vi "SQL_EDITOR_prepare_SELECT_statement.vi"(7 "nmb_of_top_rows (all)":i32, 8 "error_in":errorcluster) -> (0 "error_out":errorcluster, 3 "SELECT_statement":string)   [LabVIEW 2019]
uses:
  FGV/SQL_EDITOR_records_display/FGV_SQL_EDITOR_records_display.ctl
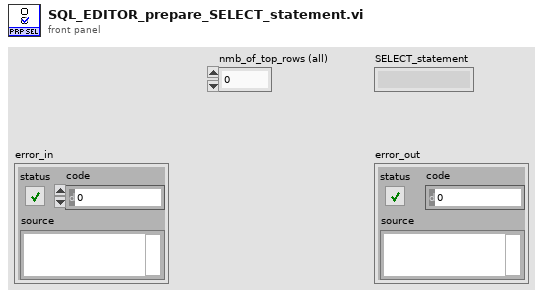
[diagram p1: front panel]
types:
  T1 = typedef "FGV_SQL_EDITOR_records_display.ctl" = enum16{"initialize", "set_table_name", "set_column_name", "set_value_to_select", "set_order_by", "set_asc_desc", "set_headers", "set_records", "get_table_name", "get_column_name", "get_value_to_select", "get_headers", "get_all_info", "record_added?", "record_inserted?", "record_edited?", "record_updated?", "record_deleted?", "discard_changes"}
  T2 = typedef "SQL_EDITOR_all_info.ctl" = cluster{"table":string, "column":string, "value_to_select":string, "order_by":string, "asc_desc":string, "headers":string[], "uneditable_columns":string[], "uneditable_columns":i32[], "editable_columns":i32[], "values_in_database":string[][], "size":cluster{"columns":i32, "SQL_rows":i32, "disp_rows":i32}, "SQL_record_states":T3[]}
  T3 = typedef "SQL_record_states.ctl" = enum16{"Equal", "Added", "Edited", "Deleted"}
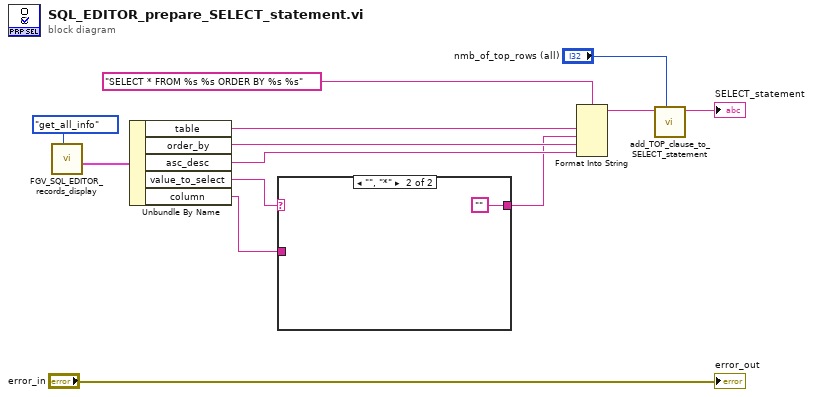
[diagram p0: block diagram]
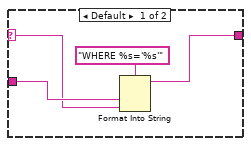
[diagram p2: hidden frame]
diagram:
  n1 = call "FGV_SQL_EDITOR_records_display.vi"("options"=FGV_SQL_EDITOR_records_display."get_all_info") -> ("all_info"=w1:T2)  [unwired: 7 in, 3 out]
  n2 = Unbundle By Name(w1) -> ("table"=w11:string, "order_by"=w13:string, "asc_desc"=w12:string, "value_to_select"=w8:string, "column"=w6:string)
  n3 = case shown="\"\", \"*\"" w8 {
    selector: w8 -> [w15 _]
    tunnel: [w14 ""] -> w7
    tunnel: w6 -> [w16 _]
    frame Default {
      n4 = Format Into String(format string="WHERE %s='%s'", w16, w15) -> (resulting string=w14:string)  [unwired: 2 in, 1 out]
    }
    frame "", "*" {
    }
  }
  n5 = Format Into String(format string="SELECT * FROM %s %s ORDER BY %s %s", w11, w7, w13, w12) -> (resulting string=w4:string)  [unwired: 2 in, 1 out]
  n6 = call "add_TOP_clause_to_SELECT_statement.vi"("nmb_of_top_rows (all)"="nmb_of_top_rows (all)", "SELECT_statement_in"=w4) -> ("SELECT_statement_out"=→"SELECT_statement":string)  [unwired: 8 in, 1 out]
  "error_out" <- "error_in"
